vi "Find and Highlight Event Frames.vi"(8 "error in":errorcluster, 10 "References":refnum<vi>[](array[refnum]), 11 "Event Name":string) -> (0 "error out":errorcluster)   [LabVIEW 2019, in "Panther Dashboard.lvlib"]
uses:
  Panther Dashboard.lvlib
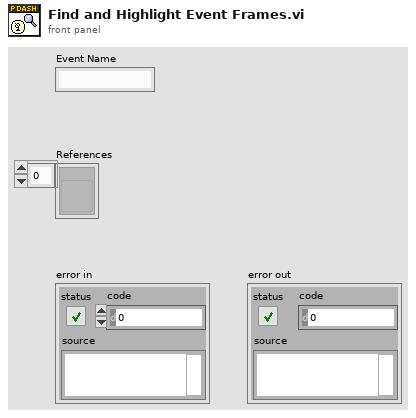
[diagram p1: front panel]
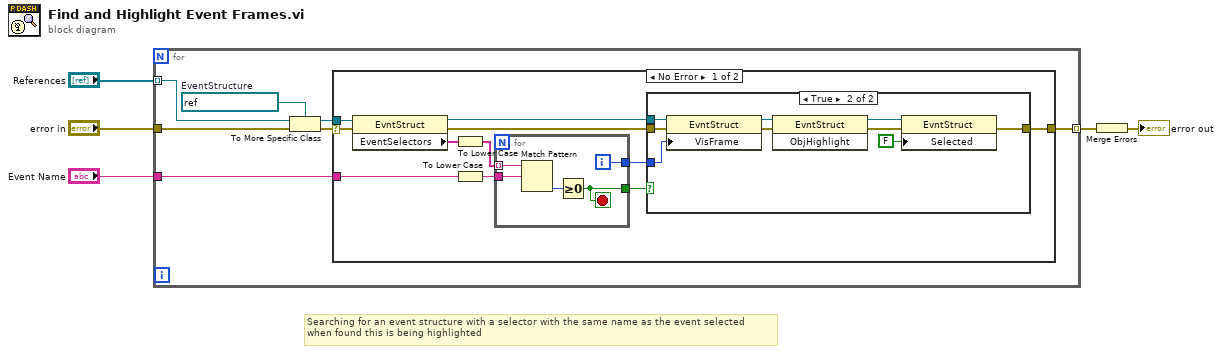
[diagram p0: block diagram]
diagram:
  # "Searching for an event structure with a selector with the same name as the event selected\nwhen found this is being highlighted"
  n1 = for {
    tunnel: "References" -> [w9] mode=indexing
    tunnel: "Event Name" -> [w6]
    tunnel: "error in" -> [w11]
    tunnel: [w10] -> w1 mode=indexing
    w8 = refnum<vi> refnum  # EventStructure
    n2 = To More Specific Class(target class=w8, reference=w9, error in=w11) -> (specific class reference=w7:refnum<vi>, error out=w12:errorcluster)
    n3 = case shown="No Error" w12 {
      selector: w12 -> [w23 _]
      tunnel: w7 -> [w18 _]
      tunnel: w6 -> [w19 _]
      tunnel: [w21 _] -> w10
      frame No Error {
        n4 = property class="EvntStruct"(reference=w18, error in=w23) -> (reference out=w15:refnum<vi>, error out=w22:errorcluster, "EventSelectors"=w20:string[])
        n5 = To Lower Case(string=w20) -> (all lower case string=w14:string[])
        n6 = To Lower Case(string=w19) -> (all lower case string=w13:string)
        n7 = for {
          tunnel: w14 -> [w38] mode=indexing
          tunnel: w13 -> [w37]
          tunnel: [w35] -> w17
          tunnel: [w34] -> w16
          i -> [w35]
          stop <- w34 stop-if-true
          n8 = Match Pattern(string=w38, regular expression=w37) -> (offset past match=w36:i32)  [unwired: 1 in, 3 out]
          n9 = Greater Or Equal To 0?(x=w36) -> (x >= 0?=w34:bool)
        }
        n10 = case shown="True" w16 {
          tunnel: w15 -> [_ w30]
          tunnel: w17 -> [_ w29]
          tunnel: w22 -> [w24 w32]
          tunnel: [w24 w27] -> w21
          frame False {
          }
          frame True {
            n11 = property class="EvntStruct"(reference=w30, error in=w32, "VisFrame"=w29) -> (reference out=w28:refnum<vi>, error out=w33:errorcluster)
            n12 = invoke class="EvntStruct" method="ObjHighlight"(reference=w28, error in=w33) -> (reference out=w26:refnum<vi>, error out=w31:errorcluster)  [unwired: 1 in, 1 out]
            n13 = property class="EvntStruct"(reference=w26, error in=w31, "Selected"=FALSE) -> (error out=w27:errorcluster)  [unwired: 1 out]
          }
        }
      }
      frame Error {
      }
    }
  }
  n14 = Merge Errors(w1) -> (→"error out":errorcluster)
